vi "SetAttributeViBoolean_ACP_SE_TOI.vi"(7 "AttributeValue (Off)":bool, 8 "error in (no error)":errorcluster {"code" format="%.0x"}, 9 "AttributeID":u32(ring)=1150129 items=["SA_ACP_AVERAGE_ENABLED"=1150129, "SA_ACP_CARRIER_REFERENCE_FREQUENCY_AUTO_ENABLED"=1150141, "SA_ACP_CARRIER_REFERENCE_LEVEL_AUTO_ENABLED"=1150143, "SA_ACP_CARRIER_REFERENCE_NUMBER_AUTO_ENABLED"=1150145, "SA_ACP_DETECTOR_TYPE_AUTO_ENABLED"=1150124, "SA_ACP_DISPLAY_BAR_GRAPH_ENABLED"=1150147, "SA_ACP_DISPLAY_WINDOWY_AUTO_SCALE_ENABLED"=1150146, "SA_ACP_FREQUENCY_PHASE_NOISE_OPTION_AUTO_ENABLED"=1150152, "SA_ACP_LIMIT_TEST_ENABLED"=1150120, "SA_ACP_MARKER_COUPLE_ENABLED"=1150236, "SA_ACP_MARKER_ENABLED"=1150238, "SA_ACP_NOISE_CORRECTION_ENABLED"=1150122, "SA_ACP_OFFSETFILTER_ENABLED"=1150166, "SA_ACP_SWEEPCOUPLING_RESOLUTION_BANDWIDTH_AUTO_ENABLED"=1150133, "SA_ACP_SWEEPCOUPLING_SWEEP_TIME_AUTO_ENABLED"=1150169, "SA_ACP_SWEEPCOUPLING_VIDEO_BANDWIDTH_AUTO_ENABLED"=1150137, "SA_SPURIOUSEMISSIONS_AVERAGE_ENABLED"=1150424, "SA_SPURIOUSEMISSIONS_DISPLAY_WINDOWY_AUTO_SCALE_ENABLED"=1150434, "SA_SPURIOUSEMISSIONS_FAST_MEASUREMENT_ENABLED"=1150426, "SA_SPURIOUSEMISSIONS_MARKER_CONTINUOUS_PEAK_SEARCH_ENABLED"=1150448, "SA_SPURIOUSEMISSIONS_MARKER_COUPLE_ENABLED"=1150441, "SA_SPURIOUSEMISSIONS_MARKER_ENABLED"=1150443, "SA_SPURIOUS_EMISSION_RANGE_TABLE_SWEEP_TYPE_AUTO_ENABLED "=1150822, "SA_THIRDORDERINTERCEPT_AVERAGE_ENABLED"=1150483, "SA_THIRDORDERINTERCEPT_LOWER_TONE_FREQUENCY_AUTO_ENABLED"=1150498, "SA_THIRDORDERINTERCEPT_SWEEPCOUPLING_BANDWIDTH_RATIO_AUTO_ENABLED"=1150494, "SA_THIRDORDERINTERCEPT_SWEEPCOUPLING_RESOLUTION_BANDWIDTH_AUTO_ENABLED"=1150487, "SA_THIRDORDERINTERCEPT_SWEEPCOUPLING_SPAN_TO_RESOLUTION_BANDWIDTH_RATIO_AUTO_ENABLED"=1150504, "SA_THIRDORDERINTERCEPT_SWEEPCOUPLING_SWEEP_TIME_AUTO_ENABLED"=1150490, "SA_THIRDORDERINTERCEPT_SWEEPCOUPLING_VIDEO_BANDWIDTH_AUTO_ENABLED"=1150492, "SA_THIRDORDERINTERCEPT_UPPER_TONE_FREQUENCY_AUTO_ENABLED"=1150499, "SA_THIRDORDERINTERCEPT_ZERO_SPAN_ENABLED"=1150506, "SA_THIRDORDERINTERCEPT_ZEROSPANSWEEPCOUPLING_RESOLUTION_BANDWIDTH_AUTO_ENABLED"=1150507, "SA_THIRDORDERINTERCEPT_ZEROSPANSWEEPCOUPLING_SWEEP_TIME_AUTO_ENABLED"=1150509], 11 "instrument handle":refnum<k15>) -> (0 "error out":errorcluster {"code" format="%.0x"}, 3 "instrument handle out":refnum<k15>)   [LabVIEW 2009, in "Keysight XSAn.lvlib"]
doc: "Sets a Boolean attribute from the instrument driver.\nThe following Attributes are supported:\n\nSA_ACP_AVERAGE_ENABLED\nSA_ACP_CARRIER_REFERENCE_FREQUENCY_AUTO_ENABLED\nSA_ACP_CARRIER_REFERENCE_LEVEL_AUTO_ENABLED\nSA_ACP_CARRIER_REFERENCE_NUMBER_AUTO_ENABLED\nSA_ACP_DETECTOR_TYPE_AUTO_ENABLED\nSA_ACP_DISPLAY_BAR_GRAPH_ENABLED\nSA_ACP_DISPLAY_WINDOWY_AUTO_SCALE_ENABLED\nSA_ACP_FREQUENCY_PHASE_NOISE_OPTION_AUTO_ENABLED\nSA_ACP_LIMIT_TEST_ENABLED\nSA_ACP_MARKER_COUPLE_ENABLED\nSA_ACP_MARKER_ENABLED\nSA_ACP_NOISE_CORRECTION_ENABLED\nSA_ACP_OFFSETFILTER_ENABLED\nSA_ACP_SWEEPCOUPLING_RESOLUTION_BANDWIDTH_AUTO_ENABLED\nSA_ACP_SWEEPCOUPLING_SWEEP_TIME_AUTO_ENABLED\nSA_ACP_SWEEPCOUPLING_VIDEO_BANDWIDTH_AUTO_ENABLED\nSA_SPURIOUSEMISSIONS_AVERAGE_ENABLED\nSA_SPURIOUSEMISSIONS_DISPLAY_WINDOWY_AUTO_SCALE_ENABLED\nSA_SPURIOUSEMISSIONS_FAST_MEASUREMENT_ENABLED\nSA_SPURIOUSEMISSIONS_MARKER_CONTINUOUS_PEAK_SEARCH_ENABLED\nSA_SPURIOUSEMISSIONS_MARKER_COUPLE_ENABLED\nSA_SPURIOUSEMISSIONS_MARKER_ENABLED\nSA_SPURIOUS_EMISSION_RANGE_TABLE_SWEEP_TYPE_AUTO_ENABLED \nSA_THIRDORDERINTERCEPT_AVERAGE_ENABLED\nSA_THIRDORDERINTERCEPT_LOWER_TONE_FREQUENCY_AUTO_ENABLED\nSA_THIRDORDERINTERCEPT_SWEEPCOUPLING_BANDWIDTH_RATIO_AUTO_ENABLED\nSA_THIRDORDERINTERCEPT_SWEEPCOUPLING_RESOLUTION_BANDWIDTH_AUTO_ENABLED\nSA_THIRDORDERINTERCEPT_SWEEPCOUPLING_SPAN_TO_RESOLUTION_BANDWIDTH_RATIO_AUTO_ENABLED\nSA_THIRDORDERINTERCEPT_SWEEPCOUPLING_SWEEP_TIME_AUTO_ENABLED\nSA_THIRDORDERINTERCEPT_SWEEPCOUPLING_VIDEO_BANDWIDTH_AUTO_ENABLED\nSA_THIRDORDERINTERCEPT_UPPER_TONE_FREQUENCY_AUTO_ENABLED\nSA_THIRDORDERINTERCEPT_ZERO_SPAN_ENABLED\nSA_THIRDORDERINTERCEPT_ZEROSPANSWEEPCOUPLING_RESOLUTION_BANDWIDTH_AUTO_ENABLED\nSA_THIRDORDERINTERCEPT_ZEROSPANSWEEPCOUPLING_SWEEP_TIME_AUTO_ENABLED"
uses:
  <instrlib>/Keysight XSAn/Keysight XSAn.lvlib
  AgXSAn.dll
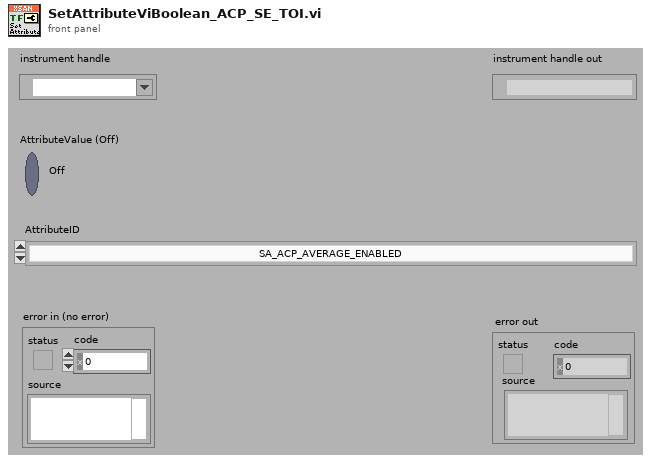
[diagram p1: front panel]
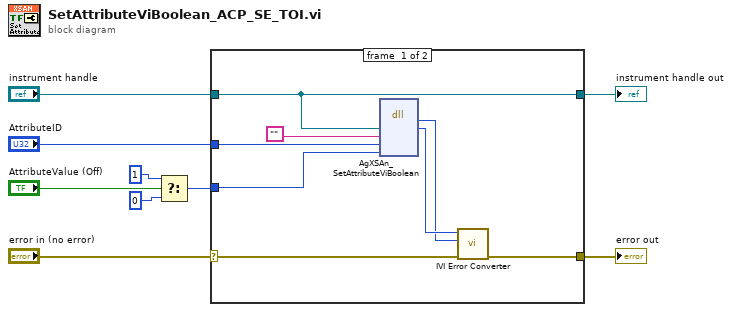
[diagram p0: block diagram]
diagram:
  n1 = Select(t=u16 1, s="AttributeValue (Off)", f=u16 0) -> (s? t:f=w2:u16)
  n2 = case shown="No Error" "error in (no error)" {
    selector: "error in (no error)" -> [w15 w19]
    tunnel: [w14 w19] -> w9
    tunnel: "instrument handle" -> [w11 w18]
    tunnel: "AttributeID" -> [w13 _]
    tunnel: w2 -> [w12 _]
    tunnel: [w11 w18] -> w1
    frame #0 {
      n3 = dll-call lib="AgXSAn**.dll" fn="AgXSAn_SetAttributeViBoolean"("Vi"=w11, "RepCapIdentifier"="", "AttributeID"=w13, "AttributeValue"=w12) -> ("return type"=w16:i32, "Vi"=w17:u32)  [unwired: 6 in, 2 out]
      n4 = call <instrlib>:"IVI Error Converter.vi"("error in (no error)"=w15, "IVI error code (0)"=w16, "instrument handle"=w17) -> ("error out"=w14:errorcluster)  [unwired: 7 in, 1 out]
    }
    frame #1 {
    }
  }
  "error out" <- w9
  "instrument handle out" <- w1
